vi "JKI.Robot.DrawRobot.vi"(8 "error in (no error)":errorcluster, 11 "JKI.Robot.SMO":refnum<class "JKI.Robot.SMO.lvclass">) -> (0 "error out":errorcluster, 2 "Picture Out":picture, 3 "JKI.Robot.SMO out":refnum<class "JKI.Robot.SMO.lvclass">)   [LabVIEW 2015, in "JKI.Robot.SMO.lvclass"]
doc: "---------------------------------------------------------------\nJKI State Machine Objects™\nhttp://jki.net/state-machine-objects/\nCopyright (C) 2005-2015, JKI <info@jki.net>\nALL RIGHTS RESERVEDJKI State Machine Objects (SMO) 1.0.0.5\nJKI - JKI\nCopyright (c) 2016, JKI"
uses:
  JKI.Robot.SMO.lvclass
  JKI.Robot.SMO.lvclass/JKI.Robot.SMO.ctl
  Private/BB9.Draw.AntiAlias.llb/BB9.Draw.Support.lvlib
panel:
  in  "Scale Factor":dbl=1.0 format="%#_13g"
  # "For instructions on how to use the JKI State Machine Objects, examples and video tutorials, visit:\nhttp://jki.net/state-machine-objects/\n\nJKI State Machine Objects™\nhttp://jki.net/state-machine-objects/\nCopyright (C) 2005-2015, JKI <info@jki.net>\nALL RIGHTS RESERVED"
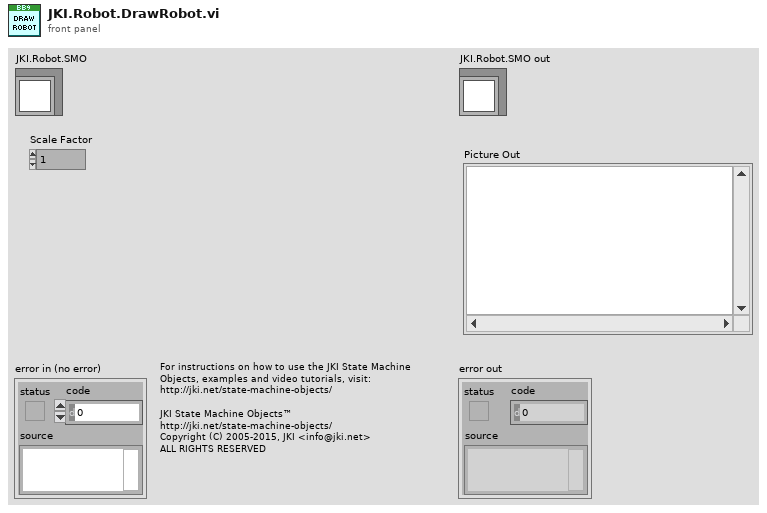
[diagram p1: front panel]
types:
  T1 = typedef "JKI.Robot.SMO.lvclass/PrivateData--Ref.ctl" = refnum<data-value>
  T2 = typedef "JKI.Robot.SMO.lvclass/PrivateData--Cluster.ctl" = cluster{"Configuration":T3, "Public Events":T4, "Robot Position":T5, "Private Events":T6}
  T3 = typedef "JKI.Robot.SMO.lvclass/Configuration--Cluster.ctl" = cluster{"Suffix":string}
  T4 = typedef "JKI.Robot.SMO.lvclass/PublicEvents--Cluster.ctl" = cluster{"Data Changed":refnum<user-event>}
  T5 = typedef "RobotPosition--Cluster.ctl" = cluster{"Claw%":dbl, "JointA":dbl, "JointB":dbl, "JointC":dbl, "JointD":dbl}
  T6 = typedef "JKI.Robot.SMO.lvclass/PrivateEvents--Cluster.ctl" = cluster{"SetGrabberPosition":refnum<user-event>, "SetJointRotation":refnum<user-event>}
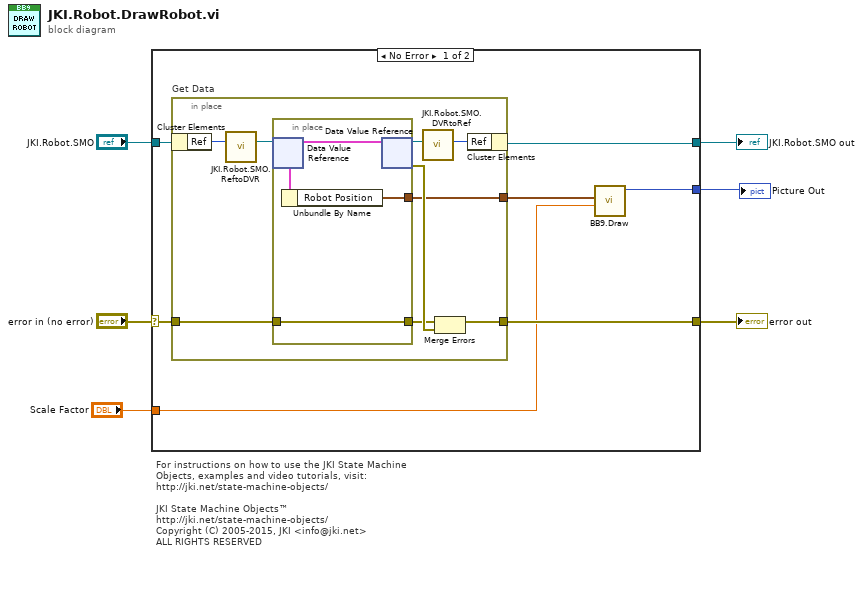
[diagram p0: block diagram]
diagram:
  # "For instructions on how to use the JKI State Machine Objects, examples and video tutorials, visit:\nhttp://jki.net/state-machine-objects/\n\nJKI State Machine Objects™\nhttp://jki.net/state-machine-objects/\nCopyright (C) 2005-2015, JKI <info@jki.net>\nALL RIGHTS RESERVED"
  n1 = case shown="No Error" "error in (no error)" {
    selector: "error in (no error)" -> [w12 w26]
    tunnel: "JKI.Robot.SMO" -> [w13 w27]
    tunnel: [w10 w26] -> w5
    tunnel: [w11 w27] -> w4
    tunnel: [w8 _] -> w2
    tunnel: "Scale Factor" -> [w7 _]
    frame No Error {
      n2 = in-place "Get Data" {
        in-place-border: w12 -> [w22]
        in-place-border: [w19] -> w10
        in-place-border: [w18] -> w9
        n3 = in-place-cluster #1(w13) -> ("Ref"=w17:u32)
        n4 = call "JKI.Robot.SMO.ReftoDVR.vi"("Ref"=w17) -> ("Ref"=w16:T1)  [unwired: 10 in]
        n5 = in-place {
          in-place-border: w22 -> [w24]
          in-place-border: [w24] -> w20
          in-place-border: [w23] -> w18
          n6 = in-place-dvr #2(w16) -> (w25:T2)  [unwired: 1 out]
          n7 = Unbundle By Name(w25) -> ("Robot Position"=w23:T5)
          n8 = in-place-dvr #2(w25) -> (w15:T1, w21:errorcluster)
        }
        n9 = call "JKI.Robot.SMO.DVRtoRef.vi"("Ref"=w15) -> ("Ref"=w14:u32)  [unwired: 10 in]
        n10 = Merge Errors(w20, w21) -> (w19:errorcluster)
        n11 = in-place-cluster #1("Ref"=w14) -> (w11:refnum<class "JKI.Robot.SMO.lvclass">)
      }
      n12 = call "BB9.Draw.vi"("Scale Factor"=w7, "Robot Position"=w9) -> ("Picture Out"=w8:picture)  [unwired: 9 in]
    }
    frame Error {
    }
  }
  "error out" <- w5
  "JKI.Robot.SMO out" <- w4
  "Picture Out" <- w2
